vi "VI Server_Decoration_Refs_FunctionalGlobal.vi"(1 "SynchRefs.Set/Get":T1, 2 "SynchRefs.IN":T2) -> (6 "SynchRefs.OUT":T2)   [LabVIEW 2020]
uses:
  VI Server_Decorations_Cluster.ctl
  toolkits_lv2020_32bit/Synchronization.llb/SynchRefs_SetGet.ctl
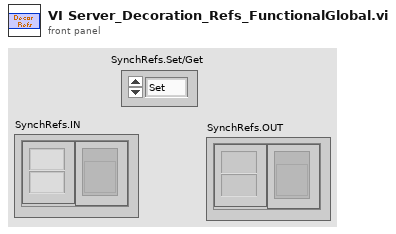
[diagram p1: front panel]
types:
  T1 = typedef "SynchRefs_SetGet.ctl" = enum16{"Set", "Get"}
  T2 = typedef "VI Server_Decorations_Cluster.ctl" = cluster{"Decoration Labels":string[], "Decorations[].Refs":refnum<vi>[]}
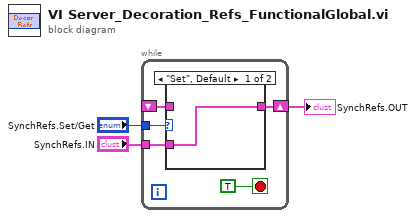
[diagram p0: block diagram]
diagram:
  n1 = while {
    tunnel: "SynchRefs.IN" -> [w6]
    tunnel: "SynchRefs.Set/Get" -> [w7]
    shift-right: [w5] -> w1
    shift-left: _ -> [w4]
    stop <- TRUE stop-if-true
    n2 = case shown="\"Set\", Default" w7 {
      tunnel: w6 -> [w9 _]
      tunnel: [w9 w10] -> w5
      tunnel: w4 -> [_ w10]
      frame "Set", Default {
      }
      frame "Get" {
      }
    }
  }
  "SynchRefs.OUT" <- w1
